vi "Defaults.vi"(1 "Do this?":bool=TRUE, 2 "Input":i64[][](array[numeric]), 3 "Absolute start time (ms)":dbl format="%.3f") -> (0 "Output":i64[][](array[numeric])=[[0, 0, 0, 0], [0, 0, 0, 0], [0, 0, 0, 0], [0, 0, 0, 0], [0, 0, 0, 0], [0, 0, 0, 0], [0, 0, 0, 0], [0, 0, 0, 0], [0, 0, 0, 0], [0, 0, 0, 0], [0, 0, 0, 0], [0, 0, 0, 0], [0, 0, 0, 0], [0, 0, 0, 0], [0, 0, 0, 0], [0, 0, 0, 0], [0, 0, 0, 0], [0, 0, 0, 0], [0, 0, 0, 0], [0, 0, 0, 0], [0, 0, 0, 0], [0, 0, 0, 0], [0, 0, 0, 1], [0, 0, 0, 1], [0, 0, 0, 1], [0, 0, 0, 1], [0, 0, 0, 1], [0, 0, 0, 1], [0, 0, 0, 1], [0, 0, 0, 1], [0, 0, 0, 1], [0, 0, 0, 1], [0, 0, 0, 1], [0, 0, 1, 0], [0, 0, 2, 0], [0, 0, 3, 0], [0, 0, 4, 0], [0, 0, 5, 1], [0, 0, 6, 1], [0, 0, 7, 1], [0, 0, 8, 0], [0, 0, 9, 1], [0, 0, 10, 0], [0, 0, 11, 0], [0, 0, 12, 0], [0, 0, 13, 0], [0, 0, 14, 1], [0, 0, 15, 1], [0, 1, 0, 1], [0, 1, 1, 1], [0, 1, 2, 0], [0, 1, 3, 0], [0, 1, 4, 0], [0, 1, 5, 1], [0, 1, 6, 0], [0, 1, 7, 0], [0, 1, 8, 0], [0, 1, 9, 0], [0, 1, 10, 1], [0, 1, 11, 0], [0, 1, 12, 1], [0, 1, 13, 0], [0, 1, 14, 0], [0, 1, 15, 0]] caption="time(ms)        port            line               value")   [LabVIEW 2017]
uses:
  globals/DIO board parameters global.vi
  globals/RIO and DAC defaults global.vi
panel:
  out "Defaults":bool[][](array[boolean])
  out "Value":bool[](array[boolean])=[FALSE, FALSE, FALSE, FALSE, FALSE, TRUE, TRUE, TRUE, FALSE, TRUE, FALSE, FALSE, FALSE, FALSE, TRUE, TRUE, TRUE, TRUE, FALSE, FALSE, FALSE, TRUE, FALSE, FALSE, FALSE, FALSE, TRUE, FALSE, TRUE, FALSE, FALSE, FALSE, FALSE, FALSE, FALSE, FALSE, FALSE, TRUE, TRUE, TRUE, FALSE, TRUE, FALSE, FALSE, FALSE, FALSE, TRUE, TRUE, TRUE, TRUE, FALSE, FALSE, FALSE, TRUE, FALSE, FALSE, FALSE, FALSE, TRUE, FALSE, TRUE, FALSE, FALSE, FALSE]
  out "Line":i32[](array[numeric])=[0, 1, 2, 3, 4, 5, 6, 7, 8, 9, 10, 11, 12, 13, 14, 15, 0, 1, 2, 3, 4, 5, 6, 7, 8, 9, 10, 11, 12, 13, 14, 15]
  out "Port":i32[](array[numeric])=[0, 0, 0, 0, 0, 0, 0, 0, 0, 0, 0, 0, 0, 0, 0, 0, 1, 1, 1, 1, 1, 1, 1, 1, 1, 1, 1, 1, 1, 1, 1, 1]
  out "Time":dbl[](array[numeric]) format="%.3f"
  # "This subVI assembles a time,port,line,value array from the default values and the absolute start time.\nThis array is then added to the Input array.  If \"Do this?\" is False, then the Output array is just the Input array."
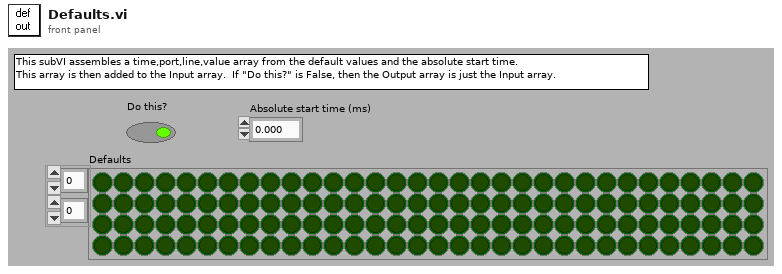
[diagram p1: front panel]
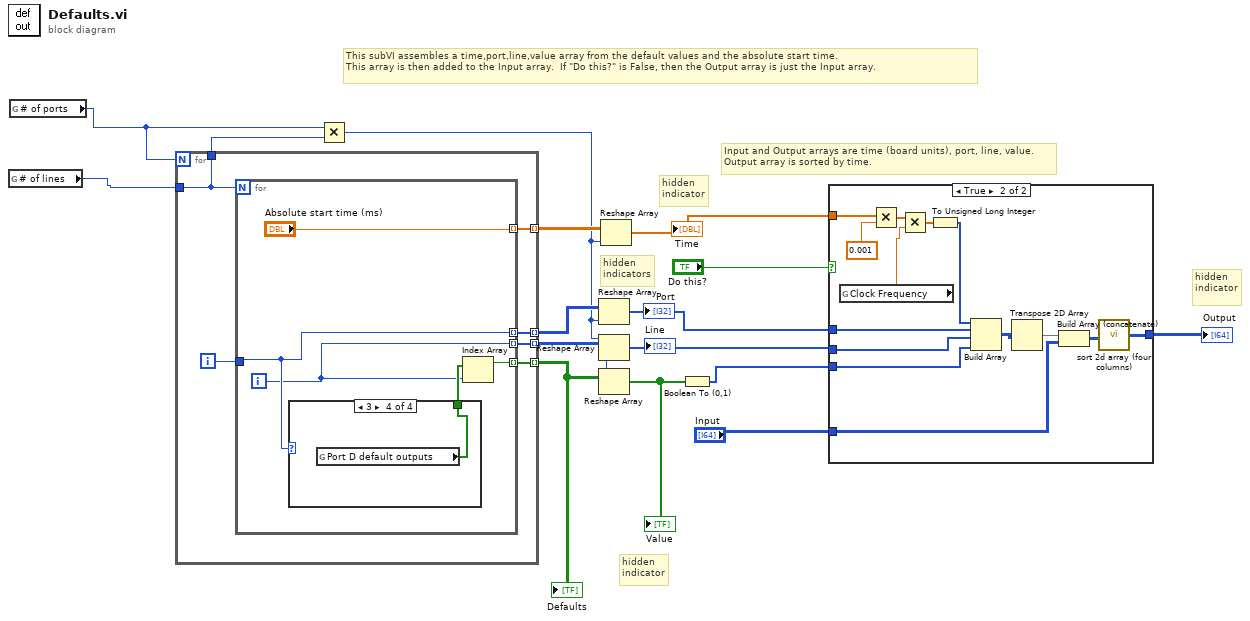
[diagram p0: block diagram]
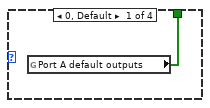
[diagram p2: hidden frame]
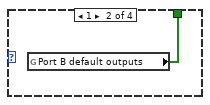
[diagram p3: hidden frame]
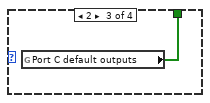
[diagram p4: hidden frame]
diagram:
  # "hidden\nindicator"
  # "hidden\nindicator"
  # "hidden\nindicator"
  # "hidden\nindicators"
  # "This subVI assembles a time,port,line,value array from the default values and the absolute start time.\nThis array is then added to the Input array.  If \"Do this?\" is False, then the Output array is just the Input array."
  # "Input and Output arrays are time (board units), port, line, value.\nOutput array is sorted by time."
  n1 = global read "DIO board parameters global.vi" "# of lines"() -> (w1:u16)
  n2 = global read "DIO board parameters global.vi" "# of ports"() -> (w2:u16)
  n3 = for {
    N: w2 -> [_]
    tunnel: [w21] -> w10 mode=indexing
    tunnel: [w20] -> w11 mode=indexing
    tunnel: [w18] -> w15 mode=indexing
    tunnel: [w19] -> w13 mode=indexing
    tunnel: [w17] -> w14
    tunnel: w1 -> [w17]
    i -> [w22]
    n4 = for {
      N: w17 -> [_]
      tunnel: [w25] -> w21 mode=indexing
      tunnel: w22 -> [w26]
      tunnel: [w23] -> w20 mode=indexing
      tunnel: [w26] -> w18 mode=indexing
      tunnel: ["Absolute start time (ms)"] -> w19 mode=indexing
      i -> [w23]
      n5 = case shown="3" w26 {
        tunnel: [w28 w29 w30 w31] -> w24
        frame 0, Default {
          n6 = global read "RIO and DAC defaults global.vi" "Port A default outputs"() -> (w28:bool[])
        }
        frame 1 {
          n7 = global read "RIO and DAC defaults global.vi" "Port B default outputs"() -> (w29:bool[])
        }
        frame 2 {
          n8 = global read "RIO and DAC defaults global.vi" "Port C default outputs"() -> (w30:bool[])
        }
        frame 3 {
          n9 = global read "RIO and DAC defaults global.vi" "Port D default outputs"() -> (w31:bool[])
        }
      }
      n10 = Index Array(array=w24, index=w23) -> (element=w25:bool)
    }
  }
  "Defaults" <- w10
  n11 = Multiply(x=w2, y=w14) -> (x*y=w12:u16)
  n12 = Reshape Array(w15, w12) -> (w3:i32[])
  "Port" <- w3
  n13 = Reshape Array(w11, w12) -> (w6:i32[])
  "Line" <- w6
  n14 = Reshape Array(w10, w12) -> (w9:bool[])
  "Value" <- w9
  n15 = Reshape Array(w13, w12) -> (w8:dbl[])
  "Time" <- w8
  n16 = Boolean To (0,1)(Boolean=w9) -> (0, 1=w4:i16[])
  n17 = case shown="True" "Do this?" {
    tunnel: "Input" -> [w32 w34]
    tunnel: [w32 w46] -> w5
    tunnel: w8 -> [_ w42]
    tunnel: w6 -> [_ w39]
    tunnel: w4 -> [_ w40]
    tunnel: w3 -> [_ w38]
    frame False {
    }
    frame True {
      n18 = global read "DIO board parameters global.vi" "Clock Frequency"() -> (w33:dbl)
      n19 = Multiply(x=w42, y=0.001) -> (x*y=w44:dbl[])
      n20 = Multiply(x=w44, y=w33) -> (x*y=w43:dbl[])
      n21 = To Unsigned Long Integer(number=w43) -> (unsigned 32bit integer=w41:u32[])
      n22 = Build Array(w41, w38, w39, w40) -> (w37:u32[][])
      n23 = Transpose 2D Array(2D array=w37) -> (transposed array=w36:u32[][])
      n24 = Build Array (concatenate)(w36, w34) -> (w35:i64[][])
      n25 = call "sort 2d array (four columns).vi"("2D array to sort"=w35) -> ("Sorted array"=w46:i64[][])
    }
  }
  "Output" <- w5
